vi "SVI-Common-VoltageCurrentConversion.vi"(8 "Current Transducer AC 0-10V In":dbl format="%#_13g", 9 "Voltage Transmitter AC 0-10V In":dbl format="%#_13g", 10 "Voltage Transmitter DC 0-10V In":dbl format="%#_13g", 11 "Current Transmitter DC 0-10V In":dbl format="%#_13g") -> (0 "Current Transducer AC 0-10V Out":dbl format="%#_13g", 1 "Voltage Transmitter AC 0-10V Out":dbl format="%#_13g", 2 "Voltage Transmitter DC 0-10V Out":dbl format="%#_13g", 3 "Current Transmitter DC 0-10V Out":dbl format="%#_13g")   [LabVIEW 2024]
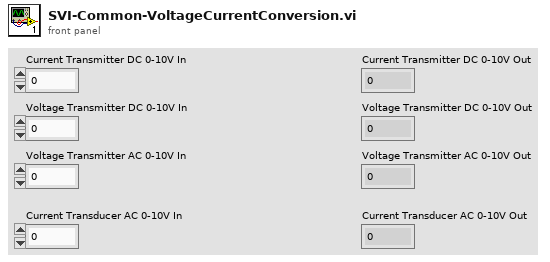
[diagram p1: front panel]
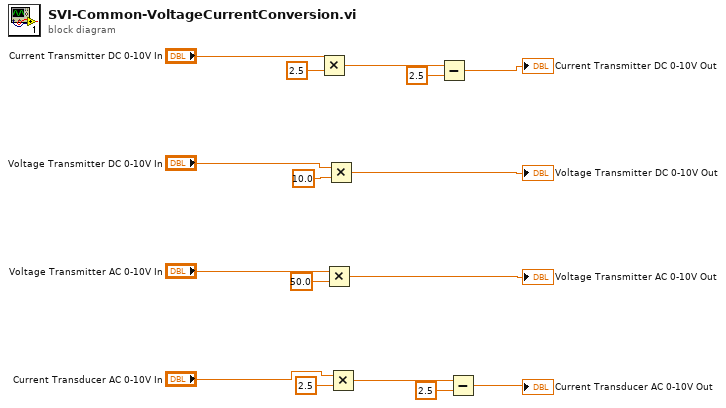
[diagram p0: block diagram]
diagram:
  n1 = Multiply(x="Current Transmitter DC 0-10V In", y=2.5) -> (x*y=w13:dbl)
  n2 = Multiply(x="Voltage Transmitter AC 0-10V In", y=50.0) -> (x*y=→"Voltage Transmitter AC 0-10V Out":dbl)
  n3 = Multiply(x="Voltage Transmitter DC 0-10V In", y=10.0) -> (x*y=→"Voltage Transmitter DC 0-10V Out":dbl)
  n4 = Multiply(x="Current Transducer AC 0-10V In", y=2.5) -> (x*y=w9:dbl)
  n5 = Subtract(x=w13, y=2.5) -> (x-y=→"Current Transmitter DC 0-10V Out":dbl)
  n6 = Subtract(x=w9, y=2.5) -> (x-y=→"Current Transducer AC 0-10V Out":dbl)
